vi "Get Waveform Streams for Data Event (CDB).vi"(8 "error in (no error)":errorcluster, 11 "registered waveform data event (CDB) in":T1) -> (0 "error out":errorcluster, 2 "WaveformStreamSpecifications":T3[](array[typedef]), 3 "registered waveform data event (CDB) out":T1)   [LabVIEW 2020, in "NI_VS Waveform Streaming Interface.lvlib"]
doc: "Returns references to all waveform stream specifications for which you previously registered for events. Wire data to the <B>registered waveform data event (DBL) in</B> input to determine the polymorphic instance to use or manually select the instance."
uses:
  <vilib>/NI VeriStand/Execution/WaveformStreaming/NI_VS Waveform Streaming Interface.lvlib
  <vilib>/NI VeriStand/Execution/WaveformStreaming/WaveformStreamSpecification.ctl
  NationalInstruments.VeriStand.ClientAPI
  <vilib>/NI VeriStand/Execution/WaveformStreaming/Registered Waveform Streams Data Event Refnum (CDB).ctl
  <vilib>/NI VeriStand/Execution/WaveformStreaming/Waveform Data Watcher Event Data (CDB).ctl
  <vilib>/NI VeriStand/Execution/WaveformStreaming/WaveformDataWatcherCDB.ctl
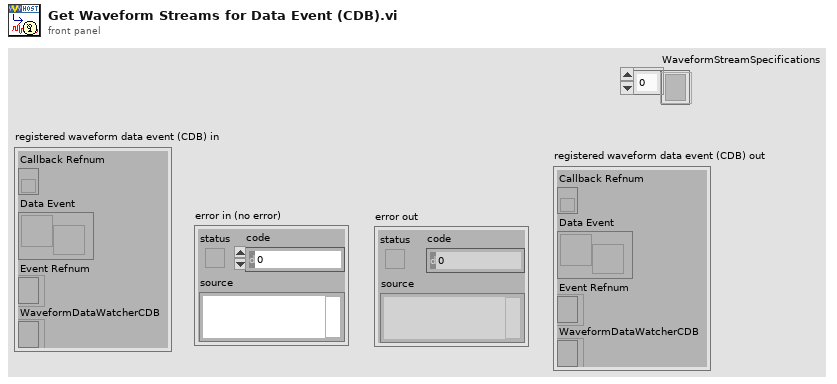
[diagram p1: front panel]
types:
  T1 = typedef "NI_VS Waveform Streaming Interface.lvlib/Registered Waveform Streams Data Event Refnum (CDB).ctl" = cluster{"Callback Refnum":refnum<k27>, "Data Event":refnum<user-event>, "Event Refnum":refnum<event-registration>, "WaveformDataWatcherCDB":T2}
  T2 = typedef "NI_VS Waveform Streaming Interface.lvlib/WaveformDataWatcherCDB.ctl" = refnum<k24>
  T3 = typedef "NI_VS Waveform Streaming Interface.lvlib/WaveformStreamSpecification.ctl" = refnum<k24>
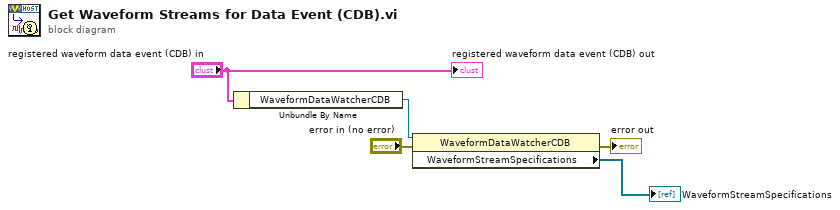
[diagram p0: block diagram]
diagram:
  n1 = Unbundle By Name("registered waveform data event (CDB) in") -> ("WaveformDataWatcherCDB"=w4:T2)
  n2 = property class="WaveformDataWatcherCDB"(reference=w4, error in="error in (no error)") -> (error out=→"error out":errorcluster, "WaveformStreamSpecifications"=→"WaveformStreamSpecifications":refnum<k24>[])  [unwired: 1 out]
  "registered waveform data event (CDB) out" <- "registered waveform data event (CDB) in"
